vi "emi_Control Enable & Visibility.vi"   [LabVIEW 2011]
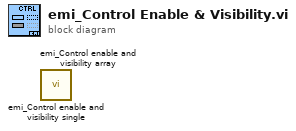
[diagram p0: block diagram]
diagram:
  n1 = call "emi_Control enable and visibility single.vi"() -> ()  [unwired: 14 in, 2 out]
  n2 = call "emi_Control enable and visibility array.vi"() -> ()  [unwired: 14 in, 2 out]
